vi "Demo VI.vi"   [LabVIEW 2020]
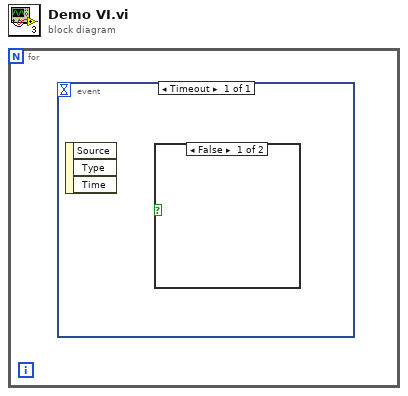
[diagram p0: block diagram]
diagram:
  n1 = for {
    n2 = event shown="[0] Timeout" {
      selector: _ -> [_]
      dyn-events: _ -> [_]
      timeout: _ -> [_]
      event Timeout {
        n3 = event-data() -> ()  [unwired: 1 in, 3 out]
        n4 = case shown="False" {
          selector: _ -> [_ _]
          frame False {
          }
          frame True {
          }
        }
      }
    }
  }
